vi "readWriteTxt.vi"() -> ()   [LabVIEW 2020]
panel:
  out "output 2":dbl
  out "output 1":dbl
  in  "2":dbl
  in  "1":dbl
  out "resulting string":string
  out "text out":string
  in  "file (use dialog)":path
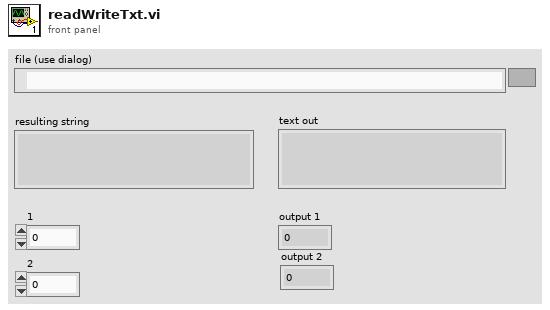
[diagram p1: front panel]
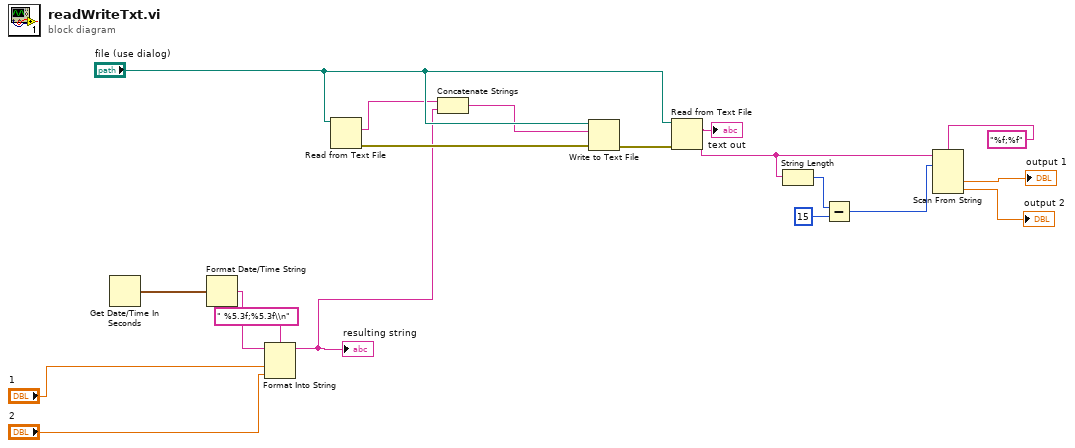
[diagram p0: block diagram]
diagram:
  n1 = Get Date/Time In Seconds() -> (seconds since 1Jan1904=w18:timestamp)
  n2 = Format Date/Time String(seconds (now)=w18) -> (date/time string=w7:string)  [unwired: 2 in]
  n3 = Format Into String(format string=" %5.3f;%5.3f\\n", initial string=w7, "1", "2") -> (resulting string=w6:string)  [unwired: 1 in, 1 out]
  "resulting string" <- w6
  n4 = Read from Text File(file (use dialog)="file (use dialog)") -> (text=w8:string, error out=w9:errorcluster)  [unwired: 3 in, 2 out]
  n5 = Concatenate Strings(w8, w6) -> (w5:string)
  n6 = Write to Text File(file (use dialog)="file (use dialog)", text=w5, error in=w9) -> (error out=w11:errorcluster)  [unwired: 1 in, 2 out]
  n7 = Read from Text File(file (use dialog)="file (use dialog)", error in=w11) -> (text=w4:string)  [unwired: 2 in, 3 out]
  "text out" <- w4
  n8 = String Length(string=w4) -> (length=w3:i32)
  n9 = Subtract(x=w3, y=15) -> (x-y=w1:i32)
  n10 = Scan From String(format string="%f;%f", input string=w4, initial scan location=w1) -> (output 1=→"output 1":dbl, output 2=→"output 2":dbl)  [unwired: 3 in, 3 out]
